vi "MAIN Modbus Test.vi"() -> ()   [LabVIEW 2019]
uses:
  <vilib>/Platform/TimedLoop/XDataNode/timing_clust.ctl
  <vilib>/Platform/TimedLoop/XDataNode/nitl_modes.ctl
  <vilib>/Platform/TimedLoop/XDataNode/wakeup.ctl
  <vilib>/FPGAPlugInAG/cRIO-9035/niLvFpga_Open_cRIO-9035.vi
  <vilib>/rvi/interface/common/dynamic/niFpgaDynamicAddResources.vi
  <vilib>/Utility/error.llb/Error Cluster From Error Code.vi
  <vilib>/rvi/errors/niLvFpgaAdjustHostInterfaceError.vi
  <vilib>/NI/Modbus Library/API/Wrapper/Create TCP Master.vi
  <vilib>/FPGAPlugInAG/Dynamic/niLvFpga_Close_Dynamic.vi
  <vilib>/platform/TimedLoop/XDataNode/XDataNode.xnode
  <vilib>/rvi/interface/nirviOpenFPGA/nirviOpenFPGA.xnode
  FPGA Bitfiles/FPGA_SENSOR.lvbitx
  <vilib>/rvi/interface/nirviReadWriteControl/nirviReadWriteControl.xnode
  <vilib>/rvi/interface/nirviCloseFPGA/nirviCloseFPGA.xnode
  <vilib>/NI/Modbus Library/API/Master/Modbus Master.lvclass
  <vilib>/Platform/TimedLoop/XDataNode/XDNodeRunTimeDep.lvlib
  NiFpgaLv.dll
  <vilib>/rvi/interface/Simulation/niFpgaSimulationCallBeginRW.vi
  <vilib>/ptbypt/NI_PtbyPt.lvlib
  <vilib>/NI/Modbus Library/API/Wrapper/API Main.lvlib
panel:
  out "Numeric":i32
  out "ma":dbl
  out "FPGA error":errorcluster
  out "connection":bool
  out "write error":errorcluster
  out "connection error":errorcluster
  out "P [MPa]":dbl format="%0.2f"
  in  "stop":bool
  out "Waveform P [MPa]":cluster{"mean":dbl, dbl}(graph)
  out "Iteration Duration":i64
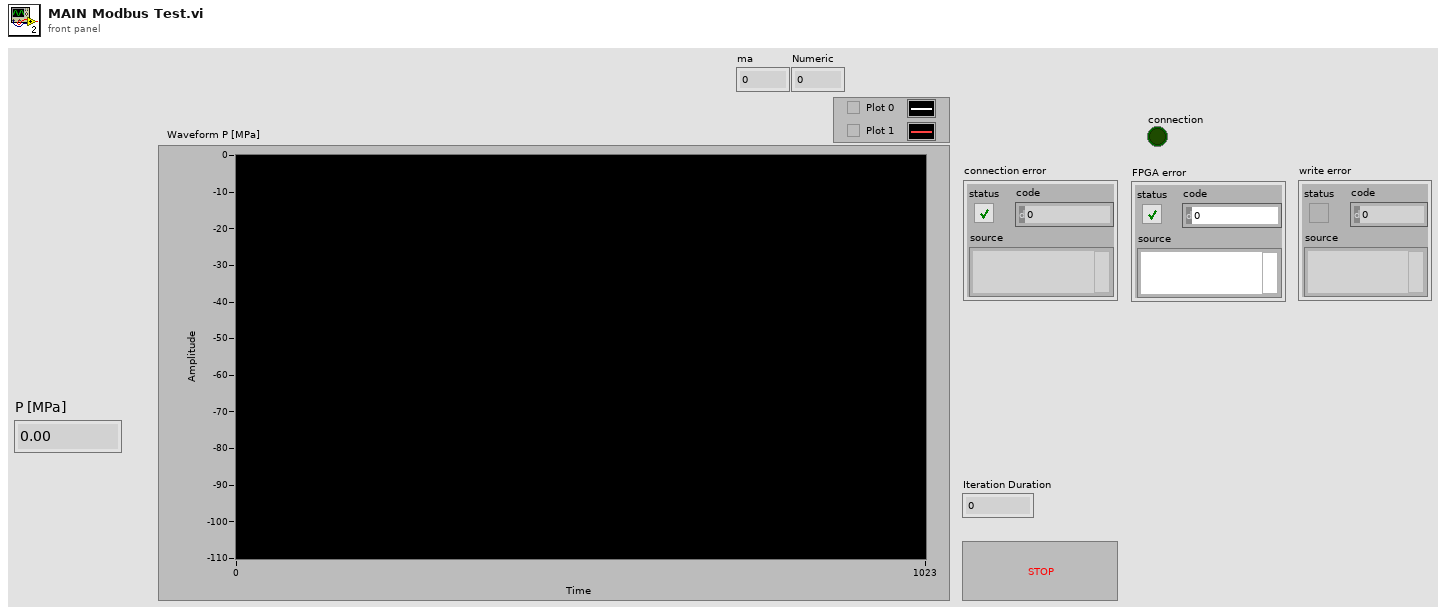
[diagram p1: front panel]
types:
  T1 = typedef "XDNodeRunTimeDep.lvlib/timing_clust.ctl" = cluster{"Expected End [f-1]":u64, "Actual End [f-1]":u64, "Finished Late? [f-1]":bool, "Expected End [i-1]":u64, "Actual End [i-1]":u64, "Finished Late? [i-1]":bool, "Expected Start [i]":u64, "Actual Start [i]":u64, "Expected Start [f]":u64, "Actual Start [f]":u64, "Source Name":string, "Structure Name":string, "Period":i64, "Deadline":i64, "Offset":i64, "Start":i64, "Priority":i32, "Timeout":i32, "Mode":T2, "Wakeup Reason":T3, "Error":errorcluster, "Source Type":string, "Secondary Source Type":string, "Global End Time":u64, "Global Start Time":u64, "Frame Duration":u64, "Iteration Duration":u64, "Assigned CPU":i32, "I/O Scan Engine Mode":u32}
  T2 = typedef "XDNodeRunTimeDep.lvlib/nitl_modes.ctl" = enum32{"No Change", "Process missed periods, maintain original phase", "Discard missed periods, maintain original phase", "Process missed periods, ignore original phase", "Discard missed periods, ignore original phase"}
  T3 = typedef "XDNodeRunTimeDep.lvlib/wakeup.ctl" = enum32{"Normal", "Aborted", "Asynchronous wakeup", "Timing source error", "Timed loop error", "Timeout"}
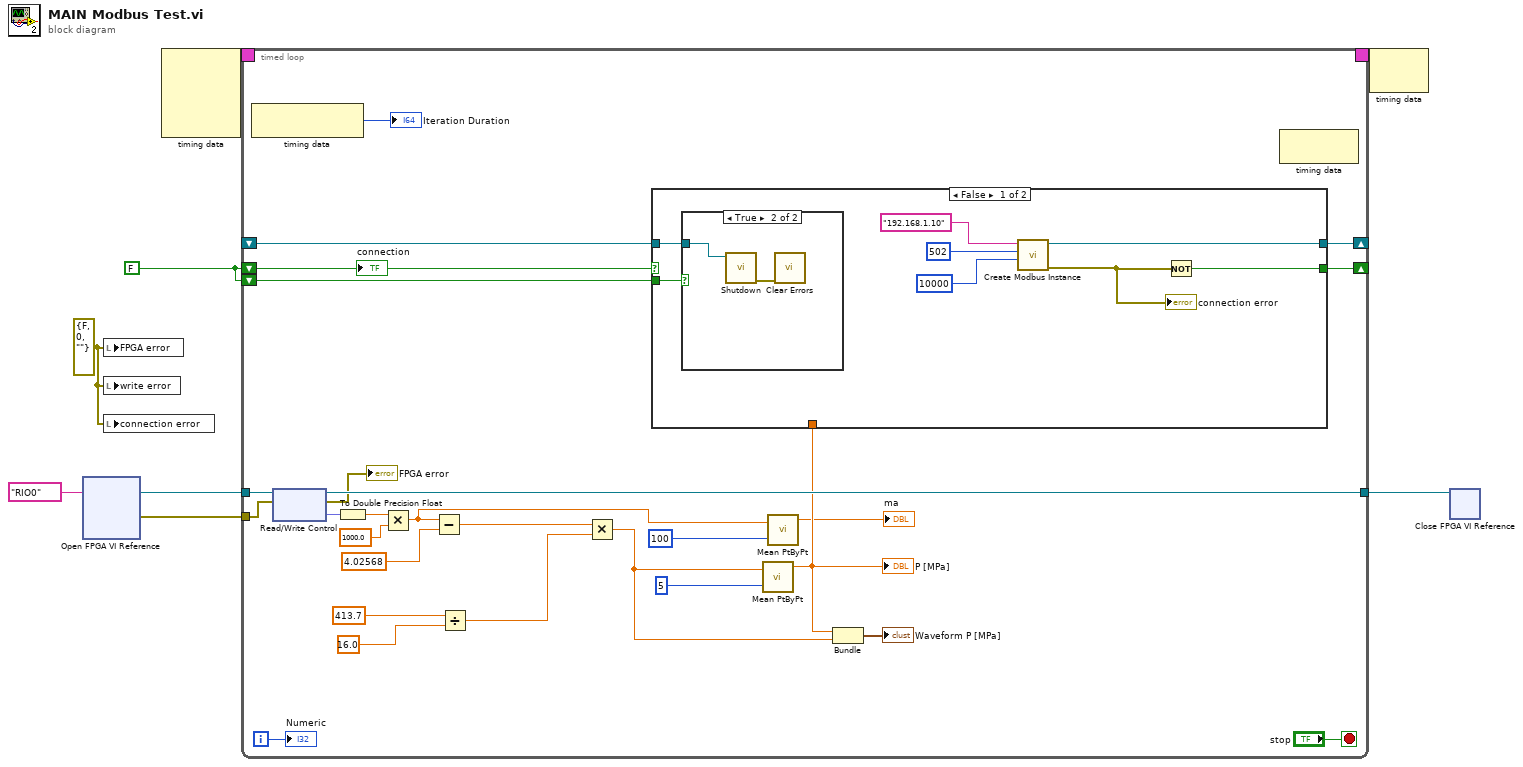
[diagram p0: block diagram]
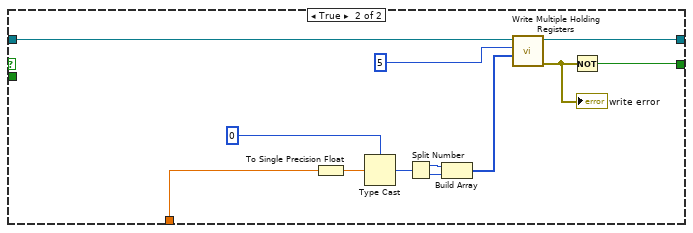
[diagram p3: hidden frame]
diagram:
  w2 = errorcluster {"status"=FALSE, "code"=0, "source"=""} ("FPGA error")
  w1 = FALSE
  n1 = xnode "Open FPGA VI Reference"("resource name"=tag "RIO0") -> ("FPGA VI Reference Out"=w5:refnum<k20>, "error out"=w3:errorcluster)  [unwired: 1 in]
  n2 = local write "FPGA error"(w2) -> ()
  n3 = local write "write error"(w2) -> ()
  n4 = local write "connection error"(w2) -> ()
  n5 = node-c288() -> (w8:T1)  [unwired: 4 in]
  n6 = timed-loop {
    timing: w8 -> [_]
    timing-out: [_] -> w7
    tunnel: w5 -> [w35]
    tunnel: [w34] -> w4
    tunnel: w3 -> [w23]
    shift-right: [w21] -> _
    shift-left: w1 -> [w22]
    shift-right: [w20] -> _
    shift-left: _ -> [w19]
    shift-left: w1 -> [w9]
    i -> [w10]
    stop <- "stop" stop-if-true
    n7 = node-c288() -> (→"Iteration Duration":i64)  [unwired: 1 in]
    n8 = xnode "Read/Write Control"("FPGA VI Reference In"=w35, "error in"=w23) -> ("FPGA VI Reference Out"=w34:refnum<k20>, "error out"=→"FPGA error":errorcluster, "AI0"=w33:fxp<+/-,21,-4>)
    n9 = To Double Precision Float(number=w33) -> (double precision float=w31:dbl)
    n10 = Multiply(x=w31, y=1000.0) -> (x*y=w12:dbl)
    n11 = Subtract(x=w12, y=4.02568) -> (x-y=w14:dbl)
    n12 = Divide(x=413.7 ("y"), y=16.0) -> (x/y=w16:dbl)
    n13 = Multiply(x=w14, y=w16) -> (x*y=w26:dbl)
    n14 = call <vilib>:"Mean PtByPt.vi"("x"=w26, "sample length"=5) -> ("mean"=w18:dbl)  [unwired: 2 in, 1 out]
    "P [MPa]" <- w18
    n15 = case shown="False" w22 {
      tunnel: [w41 w55] -> w21
      tunnel: [w40 w54] -> w20
      tunnel: w19 -> [w36 w57]
      tunnel: w18 -> [_ w52]
      tunnel: w9 -> [w37 _]
      frame False {
        n16 = case shown="True" w37 {
          tunnel: w36 -> [_ w45]
          frame False {
          }
          frame True {
            n17 = call-dynamic "Shutdown.vi"("Modbus master in"=w45) -> ("error out"=w44:errorcluster)  [unwired: 10 in]
            n18 = call <vilib>:"Clear Errors.vi"("error in (no error)"=w44) -> ()  [unwired: 5 in, 2 out]
          }
        }
        n19 = call-poly <vilib>:"Create Modbus Instance.vi"("connect timeout ms"=10000, "port (502)"=u16 502, "address"="192.168.1.10") -> ("error out"=w42:errorcluster, "TCP master instance"=w40:refnum<class "Modbus Master.lvclass">)  [unwired: 7 in]
        "connection error" <- w42
        n20 = Not(x=w42) -> (.not. x?=w41:bool)
      }
      frame True {
        n21 = To Single Precision Float(number=w52) -> (single precision float=w51:sgl)
        n22 = Type Cast(type=u32 0, x=w51) -> (*(type *) &x=w49:u32)
        n23 = Split Number(x=w49) -> (hi(x)=w48:u16, lo(x)=w47:u16)
        n24 = Build Array(w48, w47) -> (w46:u16[])
        n25 = call-dynamic "Write Multiple Holding Registers.vi"("registers to write"=w46, "starting address"=u16 5, "Modbus master in"=w57) -> ("error out"=w56:errorcluster, "Modbus master out"=w54:refnum<class "Modbus Master.lvclass">)  [unwired: 7 in]
        "write error" <- w56
        n26 = Not(x=w56) -> (.not. x?=w55:bool)
      }
    }
    n27 = call <vilib>:"Mean PtByPt.vi"("x"=w12, "sample length"=100) -> ("mean"=→"ma":dbl)  [unwired: 2 in, 1 out]
    n28 = Bundle("mean"=w18, w26) -> (→"Waveform P [MPa]":cluster{"mean":dbl, dbl})  [unwired: 1 in]
    n29 = node-c288() -> ()  [unwired: 1 in, 1 out]
    "connection" <- w22
    "Numeric" <- w10
  }
  n30 = node-c288(w7) -> ()  [unwired: 1 out]
  n31 = xnode "Close FPGA VI Reference"("FPGA VI Reference In"=w4) -> ()  [unwired: 1 in, 1 out]
